vi "dBm 2 volt.vi"(1 "dBm":dbl) -> (0 "V":dbl)   [LabVIEW 2021]
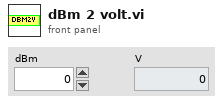
[diagram p1: front panel]
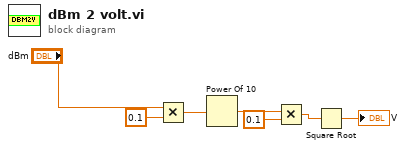
[diagram p0: block diagram]
diagram:
  n1 = Multiply(x="dBm", y=0.1) -> (x*y=w3:dbl)
  n2 = Power Of 10(x=w3) -> (10^x=w4:dbl)
  n3 = Multiply(x=w4, y=0.1) -> (x*y=w6:dbl)
  n4 = Square Root(x=w6) -> (sqrt(x)=→"V":dbl)
